vi "Configure Acquisition Bandwidth.vi"(8 "error in (no error)":errorcluster, 10 "Acquisition Bandwidth (1000000000)":i32=1000000000, 11 "VISA resource name":refnum<visa-resource-name>) -> (0 "error out":errorcluster, 3 "VISA resource name out":refnum<visa-resource-name>)   [LabVIEW 2020, in "Agilent 90000 Series.lvlib"]
doc: "Configures the bandwidth frequency control for the acquisition system."
uses:
  Agilent 90000 Series.lvlib
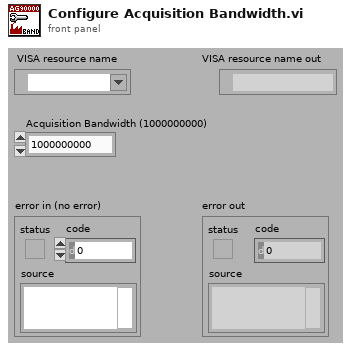
[diagram p1: front panel]
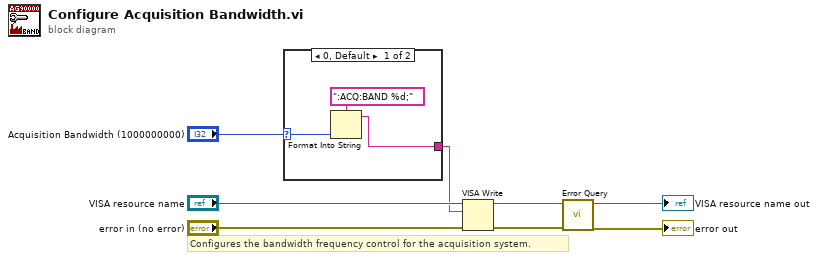
[diagram p0: block diagram]
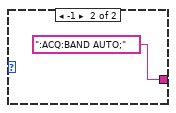
[diagram p2: hidden frame]
diagram:
  # "Configures the bandwidth frequency control for the acquisition system."
  n1 = case shown="0, Default" "Acquisition Bandwidth (1000000000)" {
    selector: "Acquisition Bandwidth (1000000000)" -> [w9 _]
    tunnel: [w10 ":ACQ:BAND AUTO;"] -> w1
    frame 0, Default {
      n2 = Format Into String(format string=":ACQ:BAND %d;", w9) -> (resulting string=w10:string)  [unwired: 2 in, 1 out]
    }
    frame -1 {
    }
  }
  n3 = VISA Write(VISA resource name="VISA resource name", write buffer=w1, error in (no error)="error in (no error)") -> (VISA resource name out=w6:refnum<visa-resource-name>, error out=w5:errorcluster)  [unwired: 1 out]
  n4 = call "Error Query.vi"("error in (no error)"=w5, "VISA resource name"=w6) -> ("error out"=→"error out":errorcluster, "VISA resource name out"=→"VISA resource name out":refnum<visa-resource-name>)  [unwired: 8 out]
